vi "Set Name Value to Default Node Clusters.vi"(8 "error in":errorcluster, 10 "Node Name":string, 11 "Clust Refnum":refnum<vi>) -> (0 "error out":errorcluster, 3 "Clust Refnum":refnum<vi>)   [LabVIEW 2025, in "Plugin XML Parser.lvlib"]
uses:
  Plugin XML Parser.lvlib
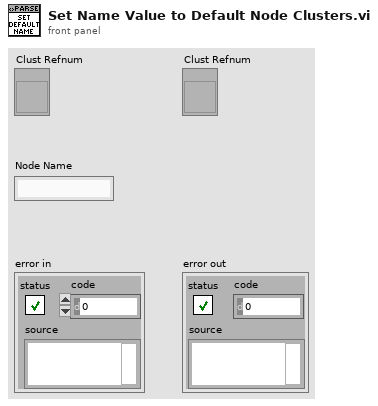
[diagram p1: front panel]
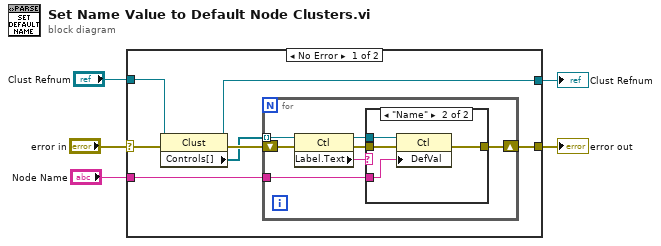
[diagram p0: block diagram]
diagram:
  n1 = case shown="No Error" "error in" {
    selector: "error in" -> [w12 w26]
    tunnel: [w10 w26] -> w4
    tunnel: "Clust Refnum" -> [w9 w25]
    tunnel: [w7 w25] -> w2
    tunnel: "Node Name" -> [w6 _]
    frame No Error {
      n2 = property class="Clust"(reference=w9, error in=w12) -> (reference out=w7:refnum<vi>, error out=w11:errorcluster, "Controls[]"=w8:refnum<vi>[])
      n3 = for {
        tunnel: w8 -> [w16] mode=indexing
        shift-right: [w17] -> w10
        shift-left: w11 -> [w19]
        tunnel: w6 -> [w14]
        n4 = property class="Ctl"(reference=w16, error in=w19) -> (reference out=w15:refnum<vi>, error out=w18:errorcluster, "Label.Text"=w13:string)
        n5 = case shown="\"Name\"" w13 {
          tunnel: w15 -> [_ w22]
          tunnel: w14 -> [_ w21]
          tunnel: w18 -> [w20 w24]
          tunnel: [w20 w23] -> w17
          frame Default {
          }
          frame "Name" {
            n6 = property class="Ctl"(reference=w22, error in=w24, "DefVal"=w21) -> (error out=w23:errorcluster)  [unwired: 1 out]
          }
        }
      }
    }
    frame Error {
    }
  }
  "Clust Refnum" <- w2
  "error out" <- w4
